vi "CenterFinderSensor.vi"(0 "VISA resource name":refnum<visa-resource-name>="COM4", 5 "controller in":refnum<k24>, 9 "Est.Center":T1 {"U" format="%#.5g"; "X" format="%#.5g"; "Y" format="%#.5g"; "Z" format="%#.5g"}, 11 "error in (no error)":errorcluster) -> (4 "VISA resource name out":refnum<visa-resource-name>, 6 "controller out":refnum<k24>, 12 "LaserCenter":T1 {"U" format="%#.5g"; "X" format="%#.5g"; "Y" format="%#.5g"; "Z" format="%#.5g"}, 13 "BoosterCenter":T1 {"U" format="%#.5g"; "X" format="%#.5g"; "Y" format="%#.5g"; "Z" format="%#.5g"}, 14 "NormalCenter":T1 {"U" format="%#.5g"; "X" format="%#.5g"; "Y" format="%#.5g"; "Z" format="%#.5g"}, 15 "error out 2":errorcluster)   [LabVIEW 2016]
uses:
  Control/Coordinate.ctl
  <vilib>/vision/NI_Vision_Development_Module.lvlib
  <vilib>/Instr/_visa.llb/VISA Configure Serial Port (Instr).vi
  <vilib>/Utility/file.llb/Read Delimited Spreadsheet (DBL).vi
  C:/Users/TTUHEP/Documents/LabVIEW/Other Models/2010/Bin/Aerotech.A3200.dll
  Other Models/2010/Bin/Aerotech.A3200.dll
panel:
  out "x/y":dbl
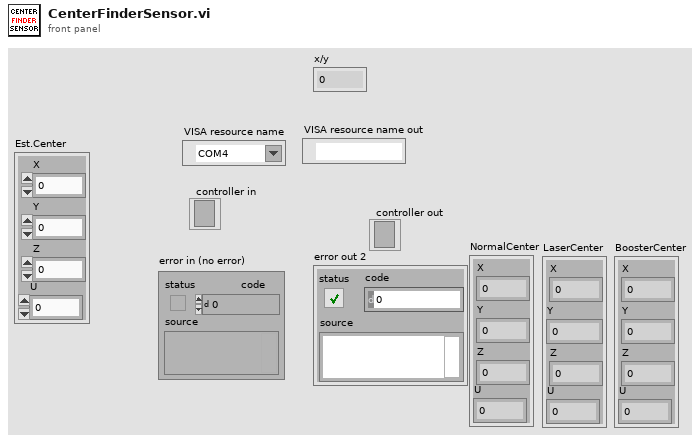
[diagram p1: front panel]
types:
  T1 = typedef "Coordinate.ctl" = cluster{"X":dbl, "Y":dbl, "Z":dbl, "U":dbl}
  T2 = enum16{"open", "replace", "create", "open or create", "replace or create", "replace or create with confirmation"}
  T3 = typedef "ControllerDiagPacket.ctl" = cluster{"Number of Diag Packets":i32, "Axes":T4[], "error":errorcluster}
  T4 = typedef "AxisDiagPacket.ctl" = cluster{"Axis Name":string, "Analog Input 0":dbl, "Analog Input 1":dbl, "Axis Fault (num)":i32, "Axis Fault (str)":string, "Axis Fault (bits)":cluster{"AmplifierFault":bool, "AmplifierTemperatureFault":bool, "CcwEndOfTravelLimitFault":bool, "CcwSoftwareLimitFault":bool, "CommunicationLostFault":bool, "CwEndOfTravelLimitFault":bool, "CwSoftwareLimitFault":bool, "EmergencyStopFault":bool, "EncoderFault":bool, "ExternalFault":bool, "FeedbackScalingFault":bool, "GantryMisalignFault ":bool, "HallSensorFault":bool, "InPositionTimeoutFault":bool, "InternalFault":bool, "MarkerSearchFault":bool, "MaxVelocityCommandFault":bool, "MissedInterruptFault":bool, "MotorTemperatureFault":bool, "None":bool, "OverCurrentFault":bool, "PositionErrorFault":bool, "PositionFeedbackFault":bool, "PowerSupplyFault":bool, "ProbeInputFault":bool, "SafeZoneFault":bool, "VelocityErrorFault":bool, "VelocityFeedbackFault":bool, "VoltageClampFault":bool}, "Axis Status (num)":i32, "Axis Status (str)":string, "Axis Status (bits)":cluster{"BacklashActive":bool, "CalibrationEnabled1D":bool, "CalibrationEnabled2D":bool, "CommandValid":bool, "DriveAbortPending":bool, "DrivePending":bool, "Enabling":bool, "GainMappingEnabled":bool, "GantryAligned":bool, "GantryRealigning":bool, "Homed":bool, "Homing":bool, "IFOVEnabled":bool, "JogGenerating":bool, "Jogging":bool, "JoystickControl":bool, "MasterSlaveControl":bool, "MotionBlocked":bool, "MotionClamped":bool, "MoveDone":bool, "None":bool, "NotVirtual":bool, "Profiling":bool, "Stability0":bool, "Stability1":bool, "TrajectoryFiltering":bool, "WaitDone":bool}, "Current Command":sgl, "Current Error":sgl, "Current Feedback":sgl, "Digital Inputs":i32, "Digital Outputs":i32, "Drive Status":i32, "Drive Status (str)":string, "Drive Status (bits)":cluster{"AccelerationPhase":bool, "AutofocusActive":bool, "BrakeOutput":bool, "CcwEndOfTravelLimitInput":bool, "CosineEncoderError":bool, "CurrentClamp":bool, "CwEndOfTravelLimitInput":bool, "DecelerationPhase":bool, "DualLoopActive":bool, "EmergencyStopInput":bool, "Enabled":bool, "EncoderClipping":bool, "GalvoCalibrationEnabled":bool, "GalvoPowerCorrection":bool, "HallAInput":bool, "HallBInput":bool, "HallCInput":bool, "HighResolutionMode":bool, "HomeLimitInput":bool, "InPosition":bool, "InPosition2":bool, "MarkerInput":bool, "MarkerLatch":bool, "MoveActive":bool, "NoMotorSupply":bool, "None":bool, "PowerLimiting":bool, "ProgrammingFlash":bool, "ProgrammingMXH":bool, "PSOHaltLatch":bool, "ServoControl":bool, "SineEncoderError":bool}, "Position Feedback Auxiliary":dbl, "Position Command":dbl, "Position Error":dbl, "Position Feedback":dbl, "Program Position Command":dbl, "Program Position Error":dbl, "Program Position Feedback":dbl, "Velocity Command":dbl, "Velocity Error":dbl, "Velocity Feedback":dbl}
  T5 = cluster{"Point 1":cluster{"X":sgl, "Y":sgl}, "Point 2":cluster{"X":sgl, "Y":sgl}}
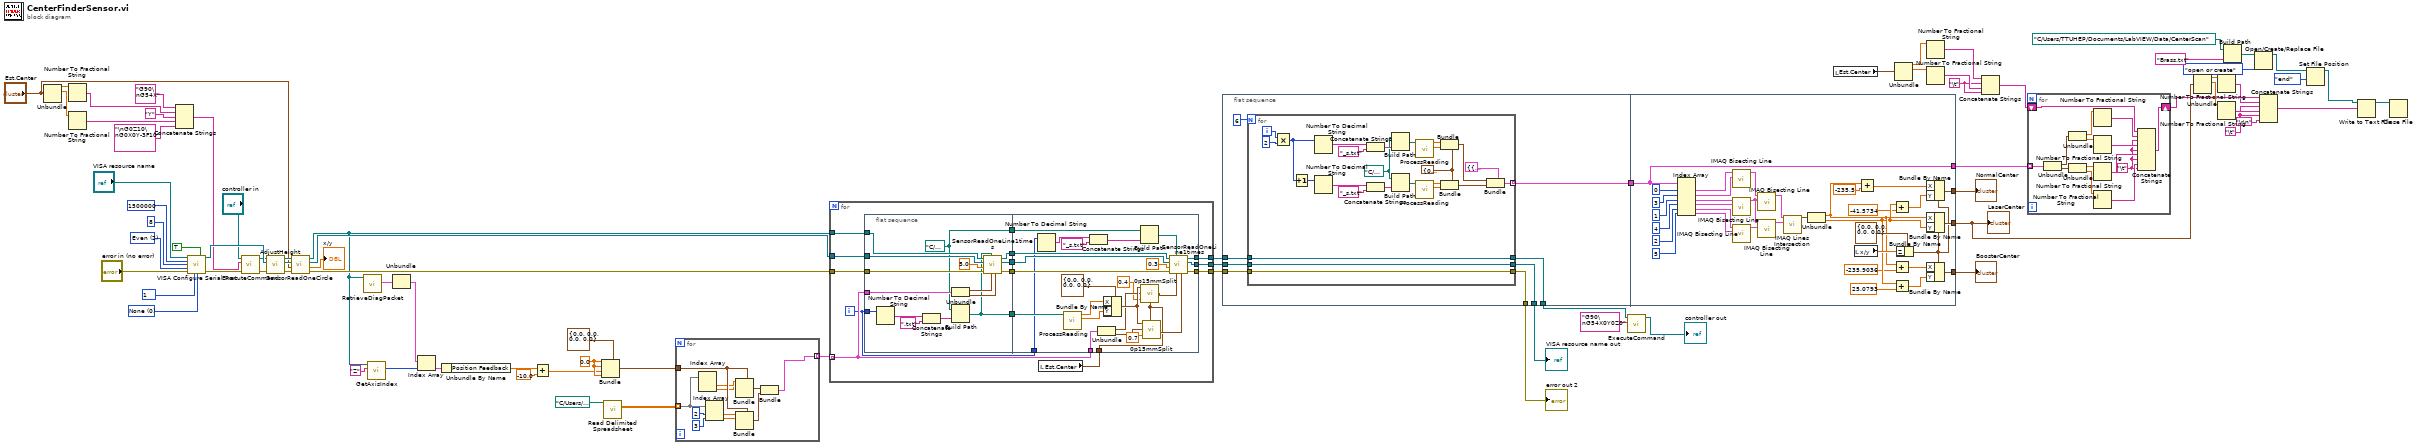
[diagram p0: block diagram]
diagram:
  w13 = "\t"
  w21 = "\t"
  w70 = u16 0 items=["None"=0, "XON/XOFF"=1, "RTS/CTS"=2, "DTR/DSR"=4] ("flow control")
  w71 = u16 10 items=["1"=10, "1.5"=15, "2.0"=20] ("stop bits")
  w72 = u16 2 items=["None", "Odd", "Even", "Mark", "Space"] ("parity")
  w76 = 0.0
  n1 = Unbundle("Est.Center") -> ("X"=w67:dbl, "Y"=w66:dbl)  [unwired: 2 out]
  n2 = Number To Fractional String(number=w67) -> (F-format string=w58:string)  [unwired: 3 in]
  n3 = Number To Fractional String(number=w66) -> (F-format string=w56:string)  [unwired: 3 in]
  n4 = Concatenate Strings("G90\nG54X", w58, "Y", w56, "\nG0Z10\nG0X0Y-3F10") -> (w49:string)
  n5 = call-poly "VISA Configure Serial Port"("VISA resource name"="VISA resource name", "Enable Termination\nChar (T)"=TRUE, "baud rate (9600)"=u32 1500000 ("baud rate"), "data bits (8)"=u16 8 ("data bits"), "parity (0:none)"=w72, "error in (no error)"="error in (no error)", "stop bits (10: 1 bit)"=w71, "flow control (0:none)"=w70) -> ("VISA resource name out"=w55:refnum<visa-resource-name>, "error out"=w54:errorcluster)  [unwired: 6 in]
  n6 = call "ExecuteCommand.vi"("error in (no error)"=w54, "Command Code"=w49, "controller in"="controller in") -> ("error out"=w51:errorcluster, "controller out"=w50:refnum<k24>)  [unwired: 6 in, 1 out]
  n7 = call "AdjustHeight.vi"("error in (no error)"=w51, "VISA resource name"=w55, 11:w50) -> ("error out"=w46:errorcluster, "VISA resource name out"=w45:refnum<visa-resource-name>, "controller out"=w47:refnum<k24>)  [unwired: 5 in, 1 out]
  n8 = call "SensorReadOneCircle.vi"("controller"=w47, "VISA resource name"=w45, "StartPoint"="Est.Center", "error out"=w46) -> ("controller out"=w40:refnum<k24>, "VISA resource name out"=w43:refnum<visa-resource-name>, "AverageReading"=→"x/y":dbl, "error out 2"=w42:errorcluster)  [unwired: 3 in]
  n9 = call "RetrieveDiagPacket.vi"("Controller In"=w40) -> ("ControllerDiagPacket"=w39:T3)  [unwired: 8 in, 2 out]
  n10 = call "GetAxisIndex.vi"("axis name"="Z", "controller in"=w40) -> ("axis index"=w37:i32)  [unwired: 7 in, 2 out]
  n11 = Unbundle(w39) -> ("Axes"=w38:T4[])  [unwired: 2 out]
  n12 = Index Array(array=w38, index=w37) -> (element=w36:T4)
  n13 = Unbundle By Name(w36) -> ("Position Feedback"=w35:dbl)
  n14 = Add(x=w35, y=-10.0) -> (x+y=w30:dbl)
  n15 = Bundle(cluster=T1 {"X"=0.0, "Y"=0.0, "Z"=0.0, "U"=0.0} ("StartPoint"), "X"=w76, "Y"=w76, "Z"=w30, "U"=w76) -> (w75:T1)
  n16 = call-poly <vilib>:"Read Delimited Spreadsheet.vi"("file path (dialog if empty)"=path "C:/Users/TTUHEP/Documents/LabVIEW/Position/CenterTest12Lines.txt") -> ("all rows"=w78:dbl[][])  [unwired: 9 in, 5 out]
  n17 = for {
    tunnel: w78 -> [w89] mode=indexing
    tunnel: w75 -> [w90]
    tunnel: [w80] -> w1 mode=indexing
    n18 = Index Array(array=w89) -> (element #1=w86:dbl, element #2=w85:dbl)  [unwired: 2 in]
    n19 = Index Array(array=w89, index #1=2, index #2=3) -> (element #1=w84:dbl, element #2=w83:dbl)
    n20 = Bundle(cluster=w90, "X"=w86, "Y"=w85) -> (w82:T1)  [unwired: 2 in]
    n21 = Bundle(cluster=w90, "X"=w84, "Y"=w83) -> (w81:T1)  [unwired: 2 in]
    n22 = Bundle("StartPoint"=w82, "StartPoint"=w81) -> (w80:cluster{"StartPoint":T1, "StartPoint":T1})  [unwired: 1 in]
  }
  n23 = for {
    tunnel: w1 -> [w95] mode=indexing
    tunnel: w40 -> [w102]
    tunnel: w43 -> [w103]
    tunnel: w42 -> [w104]
    tunnel: [w101] -> w64
    tunnel: [w100] -> w65
    tunnel: [w94] -> w63
    i -> [w92]
    n24 = flat-sequence {
      tunnel: w95 -> [w120]
      tunnel: w104 -> [w118]
      tunnel: w103 -> [w117]
      tunnel: w102 -> [w116]
      tunnel: w92 -> [w113]
      tunnel: [w109] -> w99
      tunnel: [w108] -> w98
      tunnel: [w107] -> w97
      tunnel: [w106] -> w96
      tunnel: [w105] -> w93
      tunnel: [w135] -> w100
      tunnel: [w137] -> w101
      tunnel: w99 -> [w140]
      tunnel: w98 -> [w141]
      tunnel: w97 -> [w139]
      tunnel: w96 -> [w146]
      tunnel: w95 -> [w145]
      tunnel: [w136] -> w94
      tunnel: w93 -> [w130]
      tunnel: w92 -> [w134]
      tunnel: w91 -> [w126]
      frame #0 {
        w105 = path "C:/Users/TTUHEP/Documents/LabVIEW/Data/Edge"
        n25 = Number To Decimal String(number=w113) -> (decimal integer string=w112:string)  [unwired: 1 in]
        n26 = Concatenate Strings(w112, ".txt") -> (w110:string)
        n27 = Unbundle(w120) -> ("StartPoint"=w119:T1, "StartPoint"=w115:T1)
        n28 = Build Path(base path=w105, name or relative path=w110) -> (appended path=w106:path)
        n29 = call "SensorReadOneLine1times.vi"("EndPoint"=w115, "StartPoint"=w119, "file (use dialog)"=w106, "error out"=w118, "Speed"=5.0, "VISA resource name"=w117, "controller"=w116) -> ("error out 2"=w107:errorcluster, "VISA resource name out"=w109:refnum<visa-resource-name>, "controller out"=w108:refnum<k24>)  [unwired: 2 in]
      }
      frame #1 {
        n30 = Number To Decimal String(number=w134) -> (decimal integer string=w133:string)  [unwired: 1 in]
        n31 = call "ProcessReading.vi"("file path (dialog if empty)"=w146) -> ("Y"=w142:dbl, "X"=w143:dbl)  [unwired: 9 in]
        n32 = Concatenate Strings(w133, "_s.txt") -> (w131:string)
        n33 = Unbundle(w145) -> ("StartPoint"=w124:T1, "StartPoint"=w121:T1)
        n34 = Bundle By Name(cluster=T1 {"X"=0.0, "Y"=0.0, "Z"=0.0, "U"=0.0} ("StartPoint"), "X"=w143, "Y"=w142) -> (w125:T1)
        n35 = Build Path(base path=w130, name or relative path=w131) -> (appended path=w129:path)
        n36 = call "0p15mmSplit.vi"("Est. Center"=w126, "Length"=0.4, "Direction"=w124, "RoughEdge"=w125) -> ("Start"=w128:T1)
        n37 = call "0p15mmSplit.vi"("Est. Center"=w126, "Length"=0.7, "Direction"=w121, "RoughEdge"=w125) -> ("Start"=w127:T1)
        n38 = call "SensorReadOneLine1times.vi"("EndPoint"=w127, "StartPoint"=w128, "file (use dialog)"=w129, "error out"=w139, "Speed"=0.3, "VISA resource name"=w140, "controller"=w141) -> ("error out 2"=w136:errorcluster, "VISA resource name out"=w137:refnum<visa-resource-name>, "controller out"=w135:refnum<k24>)  [unwired: 2 in]
      }
    }
    n39 = local read "Est.Center"() -> (w91:T1)
  }
  n40 = flat-sequence {
    tunnel: w65 -> [w152]
    tunnel: w64 -> [w151]
    tunnel: w63 -> [w150]
    tunnel: [w149] -> w32
    tunnel: [w148] -> w61
    tunnel: [w147] -> w60
    tunnel: [w153] -> w53
    tunnel: w53 -> [w180]
    tunnel: [w195] -> w19
    tunnel: [w183] -> w28
    tunnel: [w182] -> w52
    tunnel: [w180] -> w27
    frame #0 {
      n41 = for {
        N: 6 -> [_]
        tunnel: [w158] -> w153 mode=indexing
        tunnel: w152 -> [w156]
        tunnel: w151 -> [w157]
        tunnel: w150 -> [w155]
        tunnel: [w155] -> w147
        tunnel: [w157] -> w148
        tunnel: [w156] -> w149
        i -> [w172]
        w161 = cluster{"X":sgl, "Y":sgl} {"X"=0.0, "Y"=0.0} ("Point 1")
        w169 = path "C:/Users/TTUHEP/Documents/LabVIEW/Data/Edge"
        n42 = Multiply(x=w172, y=2) -> (x*y=w173:i32)
        n43 = Increment(x=w173) -> (x+1=w170:i32)
        n44 = Number To Decimal String(number=w173) -> (decimal integer string=w177:string)  [unwired: 1 in]
        n45 = Number To Decimal String(number=w170) -> (decimal integer string=w175:string)  [unwired: 1 in]
        n46 = Concatenate Strings(w177, "_s.txt") -> (w179:string)
        n47 = Concatenate Strings(w175, "_s.txt") -> (w168:string)
        n48 = Build Path(base path=w169, name or relative path=w179) -> (appended path=w176:path)
        n49 = Build Path(base path=w169, name or relative path=w168) -> (appended path=w167:path)
        n50 = call "ProcessReading.vi"("file path (dialog if empty)"=w176) -> ("Y"=w164:dbl, "X"=w165:dbl)  [unwired: 9 in]
        n51 = call "ProcessReading.vi"("file path (dialog if empty)"=w167) -> ("Y"=w162:dbl, "X"=w163:dbl)  [unwired: 9 in]
        n52 = Bundle(cluster=w161, "X"=w165, "Y"=w164) -> (w160:cluster{"X":sgl, "Y":sgl})
        n53 = Bundle(cluster=w161, "X"=w163, "Y"=w162) -> (w159:cluster{"X":sgl, "Y":sgl})
        n54 = Bundle(cluster=T5 {"Point 1"={"X"=0.0, "Y"=0.0}, "Point 2"={"X"=0.0, "Y"=0.0}} ("Line 1"), "Point 1"=w160, "Point 2"=w159) -> (w158:T5)
      }
    }
    frame #1 {
      n55 = Index Array(array=w180, index #1=0, index #2=3, index #3=1, index #4=4, index #5=2, index #6=5) -> (element #1=w203:T5, element #2=w207:T5, element #3=w208:T5, element #4=w209:T5, element #5=w210:T5, element #6=w204:T5)
      n56 = call "IMAQ Bisecting Line"("Line 2"=w207, "Line 1"=w203) -> ("Bisecting Line"=w211:T5)  [unwired: 8 in, 1 out]
      n57 = call "IMAQ Bisecting Line"("Line 2"=w209, "Line 1"=w208) -> ("Bisecting Line"=w212:T5)  [unwired: 8 in, 1 out]
      n58 = call "IMAQ Bisecting Line"("Line 2"=w204, "Line 1"=w210) -> ("Bisecting Line"=w213:T5)  [unwired: 8 in, 1 out]
      n59 = call "IMAQ Bisecting Line"("Line 2"=w212, "Line 1"=w211) -> ("Bisecting Line"=w205:T5)  [unwired: 8 in, 1 out]
      n60 = call "IMAQ Bisecting Line"("Line 2"=w213, "Line 1"=w212) -> ("Bisecting Line"=w206:T5)  [unwired: 8 in, 1 out]
      n61 = call "IMAQ Lines Intersection"("Line 2"=w206, "Line 1"=w205) -> ("Intersection Point"=w214:cluster{"X":sgl, "Y":sgl})  [unwired: 7 in, 2 out]
      n62 = Unbundle(w214) -> ("X"=w189:sgl, "Y"=w188:sgl)
      n63 = local read "x/y"() -> (w196:dbl)
      n64 = Add(x=w189, y=-235.5) -> (x+y=w191:dbl)
      n65 = Add(x=w188, y=-41.5734) -> (x+y=w190:dbl)
      n66 = Add(x=w189, y=-235.9036) -> (x+y=w193:dbl)
      n67 = Add(x=w188, y=25.0793) -> (x+y=w192:dbl)
      n68 = Bundle By Name(cluster=T1 {"X"=0.0, "Y"=0.0, "Z"=0.0, "U"=0.0} ("Est.Center 2"), "Z"=w196) -> (w181:T1)
      n69 = Bundle By Name(cluster=w181, "X"=w191, "Y"=w190) -> (w182:T1)
      n70 = Bundle By Name(cluster=w181, "X"=w189, "Y"=w188) -> (w195:T1)
      n71 = Bundle By Name(cluster=w181, "X"=w193, "Y"=w192) -> (w183:T1)
    }
  }
  n72 = call "ExecuteCommand.vi"("Command Code"="G90\nG54X0Y0Z0", "controller in"=w32) -> ("controller out"=→"controller out":refnum<k24>)  [unwired: 7 in, 2 out]
  n73 = local read "Est.Center"() -> (w26:T1)
  n74 = Unbundle(w26) -> ("X"=w25:dbl, "Y"=w24:dbl)  [unwired: 2 out]
  n75 = Number To Fractional String(number=w25) -> (F-format string=w23:string)  [unwired: 3 in]
  n76 = Number To Fractional String(number=w24) -> (F-format string=w22:string)  [unwired: 3 in]
  n77 = Concatenate Strings(w23, w21, w22, w21) -> (w20:string)
  n78 = for {
    tunnel: w27 -> [w228] mode=indexing
    shift-right: [w215] -> w16
    shift-left: w20 -> [w216]
    w217 = "\t"
    n79 = Unbundle(w228) -> ("Point 1"=w227:cluster{"X":sgl, "Y":sgl}, "Point 2"=w226:cluster{"X":sgl, "Y":sgl})
    n80 = Unbundle(w227) -> ("X"=w225:sgl, "Y"=w224:sgl)
    n81 = Unbundle(w226) -> ("X"=w223:sgl, "Y"=w222:sgl)
    n82 = Number To Fractional String(number=w225) -> (F-format string=w221:string)  [unwired: 3 in]
    n83 = Number To Fractional String(number=w224) -> (F-format string=w220:string)  [unwired: 3 in]
    n84 = Number To Fractional String(number=w223) -> (F-format string=w219:string)  [unwired: 3 in]
    n85 = Number To Fractional String(number=w222) -> (F-format string=w218:string)  [unwired: 3 in]
    n86 = Concatenate Strings(w216, w221, w217, w220, w217, w219, w217, w218, w217) -> (w215:string)
  }
  n87 = Unbundle(w19) -> ("X"=w18:dbl, "Y"=w17:dbl)  [unwired: 2 out]
  n88 = Number To Fractional String(number=w18) -> (F-format string=w15:string)  [unwired: 3 in]
  n89 = Number To Fractional String(number=w17) -> (F-format string=w14:string)  [unwired: 3 in]
  n90 = Build Path(base path=path "C:/Users/TTUHEP/Documents/LabVIEW/Data/CenterScan" ("file path (use dialog)"), name or relative path="Brass.txt") -> (appended path=w5:path)
  n91 = Open/Create/Replace File(file path (use dialog)=w5, operation (0:open)=T2."open or create") -> (refnum out=w10:refnum<file>)  [unwired: 4 in, 2 out]
  n92 = Concatenate Strings(w16, w15, w13, w14, w13, "\r\n") -> (w8:string)
  n93 = Set File Position(refnum=w10, from (0:start)=enum16{"start", "end", "current"}."end") -> (refnum out=w9:refnum<file>)  [unwired: 2 in, 1 out]
  n94 = Write to Text File(file (use dialog)=w9, text=w8) -> (refnum out=w7:refnum<file>)  [unwired: 2 in, 2 out]
  n95 = Close File(refnum=w7) -> ()  [unwired: 1 in, 2 out]
  "VISA resource name out" <- w61
  "error out 2" <- w60
  "LaserCenter" <- w19
  "BoosterCenter" <- w28
  "NormalCenter" <- w52
